vi "Limit AO DC.vi"(8 "error in (no error)":errorcluster, 11 "Instrument.DAQ":refnum<class "Instrument.DAQ.lvclass">) -> (0 "error out":errorcluster, 3 "Instrument.DAQ out":refnum<class "Instrument.DAQ.lvclass">)   [LabVIEW 2019, in "Instrument.Lockin.lvlib" / "Instrument.DAQ.lvclass"]
uses:
  Instrument.DAQ.lvclass
  Instrument.DAQ.lvclass/Instrument.DAQ.ctl
panel:
  # "Limit DC"
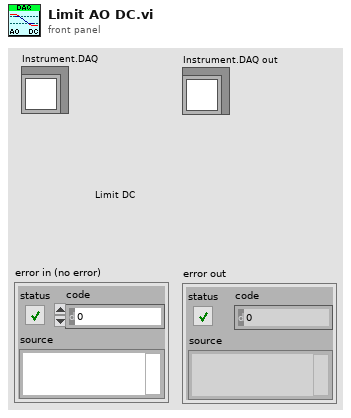
[diagram p1: front panel]
types:
  T1 = typedef "Instrument.Lockin.lvlib/Instrument.DAQ.lvclass/AO.Channel--Cluster--Array.ctl" = T2[]
  T2 = typedef "Instrument.Lockin.lvlib/Instrument.DAQ.lvclass/AO.Channel--Cluster.ctl" = cluster{"Enable?":bool, "Channel":i32, "Amplitude":dbl, "Offset":dbl, "Frequency":dbl, "Phase":dbl, "Function":T3, "Sweeping?":bool, "Limit AC":bool, "Limit DC?":bool, "Duty Cycle":bool}
  T3 = typedef "Instrument.Lockin.lvlib/Instrument.DAQ.lvclass/AO.Channel.Function--Enum.ctl" = enum16{"sine", "square", "triangle", "saw"}
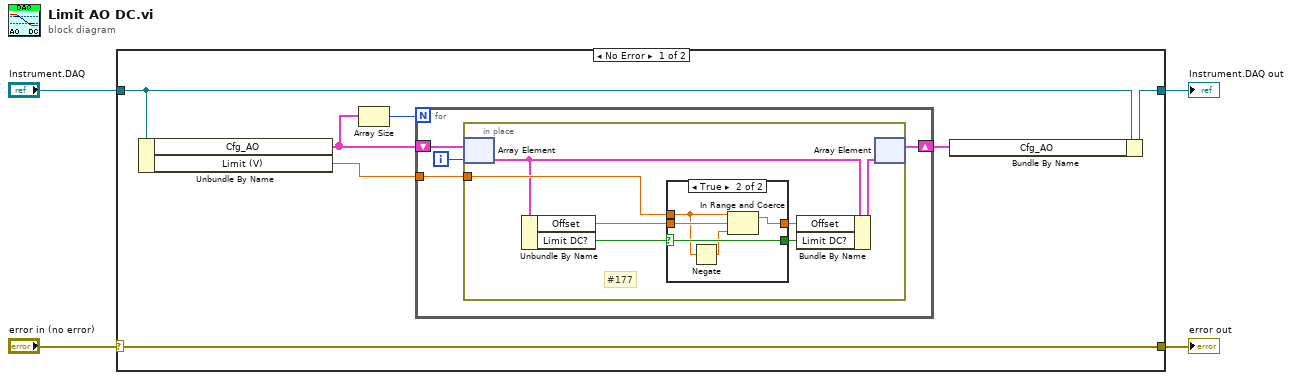
[diagram p0: block diagram]
diagram:
  n1 = case shown="No Error" "error in (no error)" {
    selector: "error in (no error)" -> [w9 w31]
    tunnel: [w11 w30] -> w4
    tunnel: "Instrument.DAQ" -> [w10 w30]
    tunnel: [w9 w31] -> w2
    frame No Error {
      n2 = Unbundle By Name(w10) -> ("Cfg_AO"=w6:T1, "Limit (V)"=w8:dbl)
      n3 = Array Size(array=w6) -> (size(s)=w7:i32)
      n4 = for {
        N: w7 -> [_]
        tunnel: w8 -> [w15]
        shift-right: [w12] -> w5
        shift-left: w6 -> [w14]
        i -> [w13]
        n5 = in-place {
          in-place-border: w15 -> [w19]
          # "#177"
          n6 = in-place-array #1(w14, w13) -> (w18:T2)
          n7 = Unbundle By Name(w18) -> ("Offset"=w22:dbl, "Limit DC?"=w16:bool)
          n8 = case shown="True" w16 {
            selector: w16 -> [w23 w27]
            tunnel: w22 -> [w24 w29]
            tunnel: w19 -> [_ w26]
            tunnel: [w24 w28] -> w21
            tunnel: [w23 w27] -> w20
            frame False {
            }
            frame True {
              n9 = Negate(x=w26) -> (-x=w25:dbl)
              n10 = In Range and Coerce(upper limit=w26, x=w29, lower limit=w25) -> (coerced(x)=w28:dbl)  [unwired: 1 out]
            }
          }
          n11 = Bundle By Name(cluster=w18, "Offset"=w21, "Limit DC?"=w20) -> (w17:T2)
          n12 = in-place-array #1(w17) -> (w12:T1)  [unwired: 1 out]
        }
      }
      n13 = Bundle By Name(cluster=w10, "Cfg_AO"=w5) -> (w11:refnum<class "Instrument.DAQ.lvclass">)
    }
    frame Error {
    }
  }
  "Instrument.DAQ out" <- w4
  "error out" <- w2
